vi "Read Logout.vi"(8 "error in (no error)":errorcluster, 11 "View Manager in":refnum<class "View Manager.lvclass">) -> (0 "error out":errorcluster, 2 "Logout":refnum<vi>, 3 "View Manager out":refnum<class "View Manager.lvclass">)   [LabVIEW 2017, in "View Manager.lvlib" / "View Manager.lvclass"]
uses:
  <vilib>/gpm_packages/@cs/User Manager App/View Manager/View Manager/View Manager.lvclass
  <vilib>/gpm_packages/@cs/User Manager App/View Manager/View Manager/View Manager.lvclass/View Manager.ctl
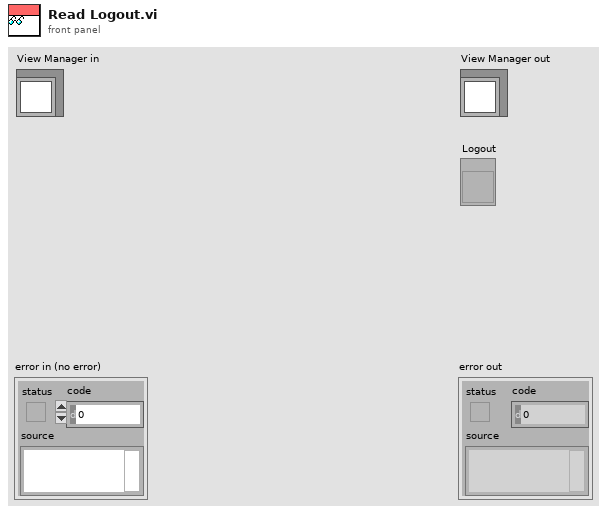
[diagram p1: front panel]
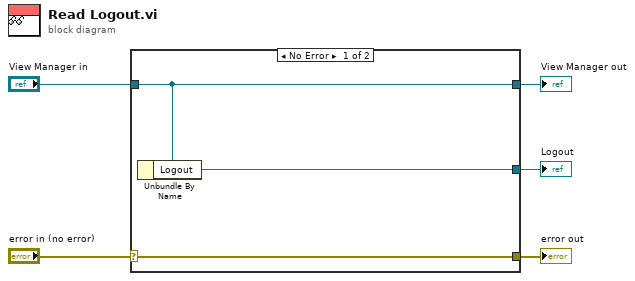
[diagram p0: block diagram]
diagram:
  n1 = case shown="No Error" "error in (no error)" {
    selector: "error in (no error)" -> [w8 w9]
    tunnel: [w8 w9] -> w4
    tunnel: [w7 w10] -> w2
    tunnel: "View Manager in" -> [w7 w10]
    tunnel: [w6 _] -> w1
    frame No Error {
      n2 = Unbundle By Name(w7) -> ("Logout"=w6:refnum<vi>)
    }
    frame Error {
    }
  }
  "error out" <- w4
  "View Manager out" <- w2
  "Logout" <- w1
